vi "VU -Set maximum velocity.vi"(7 "Action":bool, 8 "error in":errorcluster, 9 "Maximum velocity\nset":dbl format="%.2f", 10 "Axis #":i8=1 min=1 max=6 step=1, 11 "Address / Port":i16=1 min=1 max=31 step=1) -> (0 "error out":errorcluster, 1 "Query the Maximum velocity\nsetting - read":string, 2 "Axis out":i8=1 min=1 max=6 step=1, 3 "Address / Port out":i16=1 min=1 max=31 step=1)   [LabVIEW 2014]
panel:
  # "Read"
  # "Write"
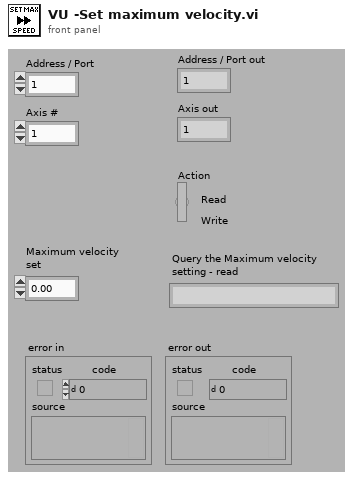
[diagram p1: front panel]
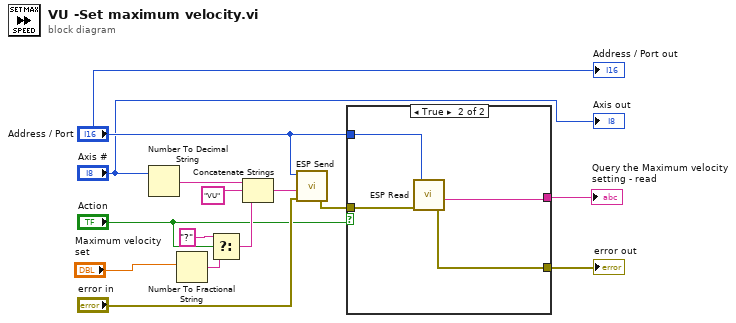
[diagram p0: block diagram]
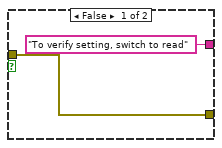
[diagram p2: hidden frame]
diagram:
  n1 = Number To Decimal String(number="Axis #") -> (decimal integer string=w14:string)  [unwired: 1 in]
  n2 = Number To Fractional String(number="Maximum velocity\nset") -> (F-format string=w10:string)  [unwired: 3 in]
  n3 = Select(t="?", s="Action", f=w10) -> (s? t:f=w11:string)
  n4 = Concatenate Strings(w14, "VU" ("Substring"), w11) -> (w12:string)
  n5 = call "ESP Send.vi"("error in"="error in", "Command String"=w12, "Address / Port"="Address / Port") -> ("error out"=w6:errorcluster)  [unwired: 3 in, 1 out]
  n6 = case shown="True" "Action" {
    tunnel: "Address / Port" -> [_ w20]
    tunnel: w6 -> [w16 w19]
    tunnel: [w16 w18] -> w5
    tunnel: ["To verify setting, switch to read" w17] -> w3
    frame False {
    }
    frame True {
      n7 = call "ESP Read.vi"("error in"=w19, "Address / Port"=w20) -> ("error out"=w18:errorcluster, "Response String"=w17:string)  [unwired: 3 in, 1 out]
    }
  }
  "error out" <- w5
  "Query the Maximum velocity\nsetting - read" <- w3
  "Address / Port out" <- "Address / Port"
  "Axis out" <- "Axis #"
